vi "Error Converter (ErrCode or Status).vi"(8 "error in (no error)":errorcluster, 11 "error code":i32) -> (0 "error out":errorcluster)   [LabVIEW 2020, in "client.lvlib"]
uses:
  client.lvlib
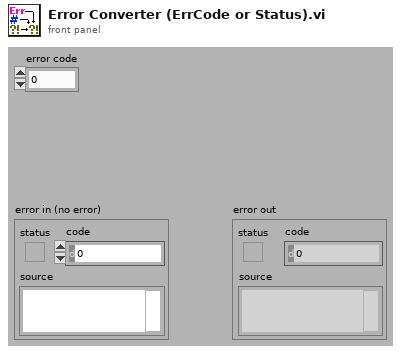
[diagram p1: front panel]
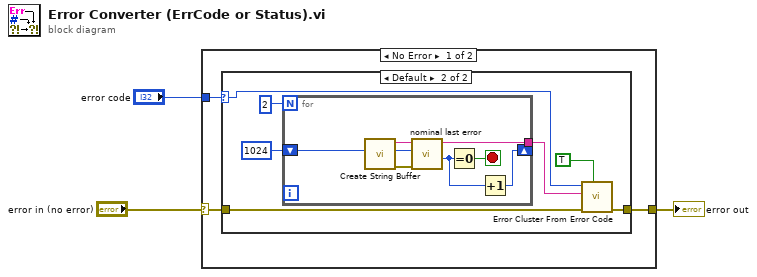
[diagram p0: block diagram]
diagram:
  n1 = case shown="No Error" "error in (no error)" {
    selector: "error in (no error)" -> [w6 w23]
    tunnel: [w4 w23] -> w2
    tunnel: "error code" -> [w5 _]
    frame No Error {
      n2 = case shown="Default" w5 {
        selector: w5 -> [_ w8]
        tunnel: w6 -> [w7 w14]
        tunnel: [w7 w13] -> w4
        frame 0 {
        }
        frame Default {
          n3 = for {
            N: 2 -> [_]
            tunnel: [w22] -> w11
            shift-right: [w19] -> _
            shift-left: 1024 -> [w16]
            stop <- w21 stop-if-true
            n4 = call "Create String Buffer.vi"("Buffer Size (1024)"=w16) -> ("error out"=w15:errorcluster, "dub Buffer Size"=w17:i32, "String Buffer"=w18:string)  [unwired: 8 in]
            n5 = call "nominal last error.vi"("error in (no error)"=w15, "cap"=w17, "buf"=w18) -> ("out_needed out"=w20:u32, "buf out"=w22:string)  [unwired: 5 in, 2 out]
            n6 = Equal To 0?(x=w20) -> (x = 0?=w21:bool)
            n7 = Increment(x=w20) -> (x+1=w19:u32)
          }
          n8 = call <vilib>:"Error Cluster From Error Code.vi"("show call chain? (False)"=TRUE, "error in (no error)"=w14, "error message (\"\")"=w11, "error code (0)"=w8) -> ("error out"=w13:errorcluster)  [unwired: 5 in]
        }
      }
    }
    frame Error {
    }
  }
  "error out" <- w2
